vi "26进制转10进制.vi"(1 "26进制":string) -> (0 "十进制":u16)   [LabVIEW 2020, in "OperateExcel.lvlib"]
uses:
  OperateExcel.lvlib
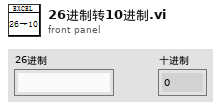
[diagram p1: front panel]
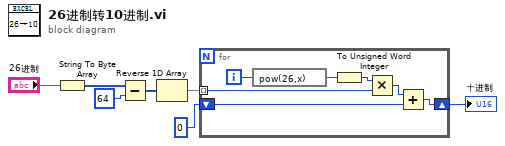
[diagram p0: block diagram]
diagram:
  n1 = String To Byte Array(string="26进制") -> (unsigned byte array=w1:u8[])
  n2 = Subtract(x=w1, y=u8 64) -> (x-y=w5:u8[])
  n3 = Reverse 1D Array(array=w5) -> (reversed array=w4:u8[])
  n4 = for {
    tunnel: w4 -> [w9] mode=indexing
    shift-right: [w13] -> w2
    shift-left: u16 0 -> [w12]
    i -> [w11]
    n5 = expression code="pow(26,x)"(w11) -> (w10:i32)
    n6 = To Unsigned Word Integer(number=w10) -> (unsigned 16bit integer=w8:u16)
    n7 = Multiply(x=w8, y=w9) -> (x*y=w14:u16)
    n8 = Add(x=w14, y=w12) -> (x+y=w13:u16)
  }
  "十进制" <- w2
